vi "Actor Core.vi"(8 "error in":errorcluster, 11 "SM EOL Station Actor in":refnum<class "OPC Server.lvclass">) -> (0 "error out":errorcluster, 3 "Actor out":refnum<class "Actor.lvclass">)   [LabVIEW 2021, in "OPC Server.lvlib" / "OPC Server.lvclass"]
doc: "(<B>Filename</B>: Actor Framework.lvlib:Actor.lvclass:Actor Core.vi)\n\nReceives messages to the actor, reacts to them, and initiates any error handling that may shut the actor down.\n\nDescendant classes may override this VI to append parallel tasks for the actor to complete while it handles messages. Overrides use the Call Parent Class Method node."
uses:
  OPC Server.lvclass
  C:/Program Files/National Instruments/LabVIEW 2021/vi.lib/ActorFramework/Actor/Actor.lvclass
  <vilib>/ActorFramework/Actor/Actor.lvclass
  <vilib>/Utility/miscctls.llb/LVComboBoxStrsAndValuesArrayTypeDef.ctl
  OPC Server.lvclass/OPC Server.ctl
  <vilib>/ActorFramework/Actor/Actor.lvclass/Actor.ctl
  <vilib>/ActorFramework/Message Enqueuer/Message Enqueuer.lvclass/Message Enqueuer.ctl
  OPC Server Messages/Select online Station Msg/Select online Station Msg.lvclass/Select online Station Msg.ctl
  <vilib>/ActorFramework/Message Enqueuer/Init from Existing Queue.vi
  <vilib>/ActorFramework/Message Enqueuer/Enqueue.vi
  OPC Server Messages/Launch New Station Msg/Launch New Station Msg.lvclass
  C:/Program Files/National Instruments/LabVIEW 2021/vi.lib/ActorFramework/Message/Message.lvclass
  OPC Server Messages/Enable New Station Msg/Enable New Station Msg.lvclass
  OPC Server Messages/Select online Station Msg/Select online Station Msg.lvclass
  <vilib>/ActorFramework/Stop Msg/Stop Msg.lvclass
  OPC Server Messages/Stop OPC UA Msg/Stop OPC UA Msg.lvclass
  <vilib>/ActorFramework/Message Priority Queue/Priority Enqueue.vi
  <vilib>/ActorFramework/Message Enqueuer/Message Enqueuer.lvclass
panel:
  out "Station Enable":string
  in  "Online Stations":string(combo)
  out "Connected?":bool
  in  "Create Station":bool
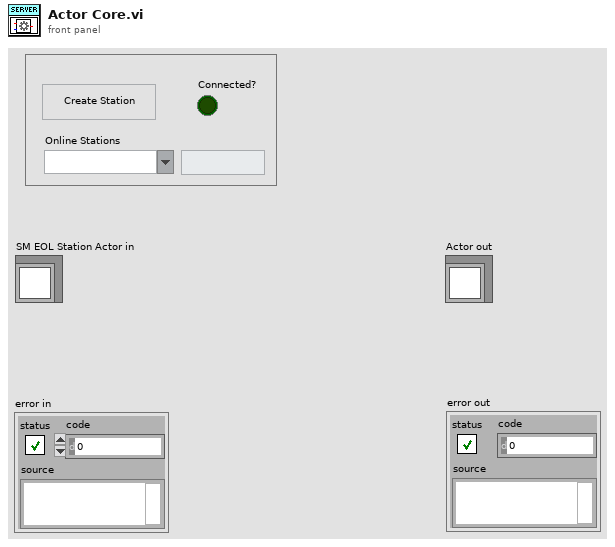
[diagram p1: front panel]
types:
  T1 = enum8{"Enabled", "Disabled", "Disabled and Grayed Out"}
  T2 = typedef "LVComboBoxStrsAndValuesArrayTypeDef.ctl" = cluster{"String":string, "Value":string}[]
  T3 = enum32{"Invalid", "Standard", "Closed", "Hidden", "Minimized", "Maximized"}
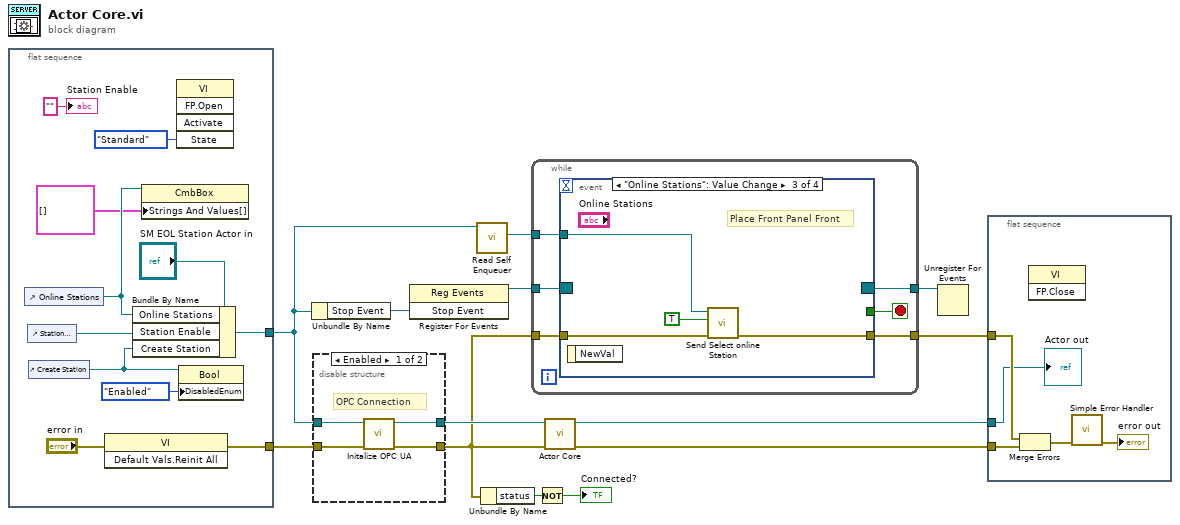
[diagram p0: block diagram]
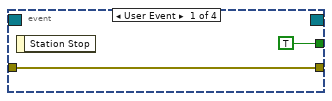
[diagram p3: hidden frame]
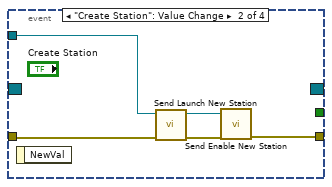
[diagram p4: hidden frame]
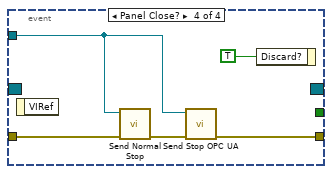
[diagram p5: hidden frame]
diagram:
  n1 = flat-sequence {
    tunnel: [w23] -> w5
    tunnel: [w20] -> w6
    frame #0 {
      n2 = control-ref of="Online Stations"() -> (w19:refnum<vi>)
      n3 = control-ref of="Station Enable"() -> (w15:refnum<vi>)
      n4 = control-ref of="Create Station"() -> (w17:refnum<vi>)
      n5 = invoke class="VI" method="Default Vals.Reinit All"(error in="error in") -> (error out=w23:errorcluster)  [unwired: 2 in, 2 out]
      n6 = Bundle By Name(cluster="SM EOL Station Actor in", "Online Stations"=w19, "Station Enable"=w15, "Create Station"=w17) -> (w20:refnum<class "OPC Server.lvclass">)
      n7 = property class="CmbBox"(reference=w19, "Strings And Values[]"=T2 [] ("Strings And Values []")) -> ()  [unwired: 1 in, 2 out]
      n8 = invoke class="VI" method="FP.Open"("State"=T3."Standard") -> ()  [unwired: 4 in, 5 out]
      n9 = property class="Bool"(reference=w17, "DisabledEnum"=T1."Enabled" ("Disabled")) -> ()  [unwired: 1 in, 2 out]
      "Station Enable" <- "" ("Station Enable")
    }
  }
  n10 = Unbundle By Name(w6) -> ("Stop Event"=w13:refnum<user-event>)
  n11 = disable-structure shown="Enabled" {
    disable-tunnel: w6 -> [w28 w30]
    disable-tunnel: w5 -> [w27 w29]
    disable-tunnel: [w26 w30] -> w4
    disable-tunnel: [w25 w29] -> w3
    frame Enabled {
      # "OPC Connection"
      n12 = call "Initalize OPC UA.vi"("error in (no error)"=w27, "SM EOL Station Actor in"=w28) -> ("error out"=w25:errorcluster, "SM EOL Station Actor out"=w26:refnum<class "OPC Server.lvclass">)  [unwired: 8 in]
    }
    frame Disabled {
    }
  }
  n13 = register-events(w13) -> (reference out=w12:refnum<event-registration>)  [unwired: 2 in, 1 out]
  n14 = call <vilib>:"Read Self Enqueuer.vi"("Actor"=w6) -> ("Self Enqueuer"=w11:refnum<class "Message Enqueuer.lvclass">)  [unwired: 10 in]
  n15 = Unbundle By Name(w3) -> ("status"=w7:bool)
  n16 = while {
    tunnel: w12 -> [w36]
    tunnel: [w35] -> w9
    tunnel: w11 -> [w34]
    tunnel: [w32] -> w10
    tunnel: w3 -> [w31]
    stop <- w33 stop-if-true
    n17 = event shown="[2] \"Online Stations\": Value Change" {
      selector: w36 -> [_ _ _ _]
      dyn-events: [_ _ _ _] -> w35
      timeout: _ -> [_ _ _ _]
      tunnel: w34 -> [_ w43 w46 w49]
      tunnel: [TRUE ("Discard?") _ _ _] -> w33
      tunnel: [w37 w39 w45 w50] -> w32
      tunnel: w31 -> [w37 w42 w47 w51]
      event User Event {
        n18 = event-data() -> ()  [unwired: 1 in, 1 out]
      }
      event "Create Station": Value Change {
        n19 = event-data() -> ()  [unwired: 1 in, 1 out]
        n20 = call "Send Launch New Station.vi"("error in (no error)"=w42, "Message Enqueuer"=w43) -> ("error out"=w40:errorcluster, "Message Enqueuer out"=w41:refnum<class "Message Enqueuer.lvclass">)  [unwired: 8 in]
        n21 = call "Send Enable New Station.vi"("error in (no error)"=w40, "Message Enqueuer"=w41) -> ("error out"=w39:errorcluster)  [unwired: 8 in, 1 out]
      }
      event "Online Stations": Value Change {
        # "Place Front Panel Front"
        n22 = event-data() -> ()  [unwired: 1 in, 1 out]
        n23 = call "Send Select online Station.vi"("error in (no error)"=w47, "FP Frontmost"=TRUE, "Message Enqueuer"=w46) -> ("error out"=w45:errorcluster)  [unwired: 7 in, 1 out]
      }
      event Panel Close? {
        n24 = event-data() -> ()  [unwired: 1 in, 1 out]
        n25 = call <vilib>:"Send Normal Stop.vi"("error in (no error)"=w51, "Message Enqueuer"=w49) -> ("error out"=w48:errorcluster)  [unwired: 9 in]
        n26 = call "Send Stop OPC UA.vi"("error in (no error)"=w48, "Message Enqueuer"=w49) -> ("error out"=w50:errorcluster)  [unwired: 8 in, 1 out]
        n27 = event-data("Discard?"=TRUE) -> ()  [unwired: 1 in, 1 out]
      }
    }
  }
  n28 = Not(x=w7) -> (.not. x?=→"Connected?":bool)
  n29 = call-parent "Actor Core.vi"("error in"=w3, "Actor in"=w4) -> ("error out"=w1:errorcluster, "Actor out"=w2:refnum<class "Actor.lvclass">)  [unwired: 8 in]
  n30 = Unregister For Events(event registration refnum=w9) -> ()  [unwired: 1 in, 1 out]
  n31 = flat-sequence {
    tunnel: w10 -> [w57]
    tunnel: w2 -> [w56]
    tunnel: w1 -> [w55]
    frame #0 {
      n32 = Merge Errors(w57, w55) -> (w54:errorcluster)
      n33 = invoke class="VI" method="FP.Close"() -> ()  [unwired: 3 in, 3 out]
      n34 = call <vilib>:"Simple Error Handler.vi"("error in (no error)"=w54) -> ("error out"=→"error out":errorcluster)  [unwired: 4 in, 4 out]
      "Actor out" <- w56
    }
  }
